vi "FPGA_main_v2.vi"() -> ()   [LabVIEW 2018]
doc: "FPGA main VI for AI input and output.\n\nSamples at 100 kHz and downsamples to 1 kHz."
uses:
  <vilib>/rvi/Emulation/niFpgaGetClockAttributes.vi
  <vilib>/rvi/Emulation/niFpgaSctlEmulationGetInTimedLoop.vi
  <vilib>/rvi/Emulation/niFpgaEmulationReportErrorSimple.vi
  <vilib>/rvi/eio/common/nirviEmuTemplateMethod_errors.vi
  <vilib>/rvi/Emulation/niFpgaEmulationIsFPGAContextNoSignature.vi
  <vilib>/rvi/errors/niFpgaSetErrorForExecOnDevCompSimple.vi
  <vilib>/rvi/eio/common/nirviEmuReportErrorAndStop.vi
  <vilib>/rvi/DataTransferAndStorage/Container/Common/niFpgaContainerGetUniqueNameForEmu.vi
  <vilib>/rvi/FIFO/Fifo_Resource/nirvififoEmulationSetSize.vi
  <vilib>/rvi/FIFO/Fifo_Resource/nirviFifoEmulationQueueMgr.vi
  <instcachedir>/0/nirviFifoEmulationQueueMgr_E5CAEC123FF24DC58D834DCA3CDAA9B5.lvgen/nirviFifoEmulationQueueMgr_E5CAEC123FF24DC58D834DCA3CDAA9B5_003.vi
  <vilib>/rvi/FIFO/Fifo_Resource/nirvififoEmulationDetermineInputValidOut.vi
  <vilib>/rvi/FIFO/Fifo_Resource/nirvififoEmulationCreateLock.vi
  <vilib>/rvi/Emulation/niFpgaProcessEmulError.vi
  <vilib>/rvi/FIFO/Fifo_Resource/nirvififoEmulationObtainLock.vi
  <vilib>/rvi/FIFO/Fifo_Resource/nirvififoEmulationReleaseLock.vi
  <vilib>/rvi/occurrence/nirviWaitOnOccurrenceBase.vi
  <vilib>/rvi/errors/nirviReportUnexpectedCaseInternalError.vi
  <vilib>/rvi/errors/nirviReportUnexpectedCaseInternalError (U32).vi
  <vilib>/rvi/Emulation/niFpgaCriticalErrorInLSC.vi
  <vilib>/Utility/error.llb/Clear Errors.vi
  <vilib>/eio/EIONode/EIONode.xnode
  <vilib>/rvi/DataTransferAndStorage/Container/XNode/niFpgaContainer.xnode
  <vilib>/rvi/FIFO/Fifo_Resource/nirvififoEmulationWrite.vi
  <vilib>/rvi/Analysis/measure/butterworth/XNode/niFpgaButterworthFilter.xnode
  <vilib>/rvi/FIFO/Fifo_Resource/nirvififoEmulationRead.vi
  Components/FPGA functions/FPGA functions.lvlib
panel:
  in  "Count(uSec)":u8=8 caption="I/O sample time (us)"
  out "LPF loop rate (us)":u8
  out "ConnectorC/AI0":fxp<+/-,16,1>
  out "Signal I/O loop rate (us)":u8
  in  "ConnectorC/AO0":i16
  # "Inputs"
  # "Sampling time"
  # "Filtered AI"
  # "For each additional bit of resolution, the signal must be oversampled by a factor of four:\nf_os = 4^w f_s \nwhere w is the number of additional bits of resolution desired, f_s is the original sampling frequency requirement, and f_os is the oversampling frequency\n\nhttp://www.cypress.com/file/236481/download"
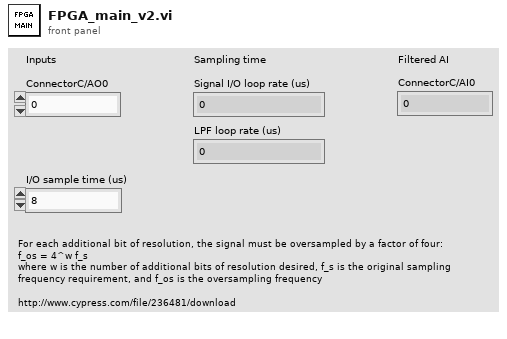
[diagram p1: front panel]
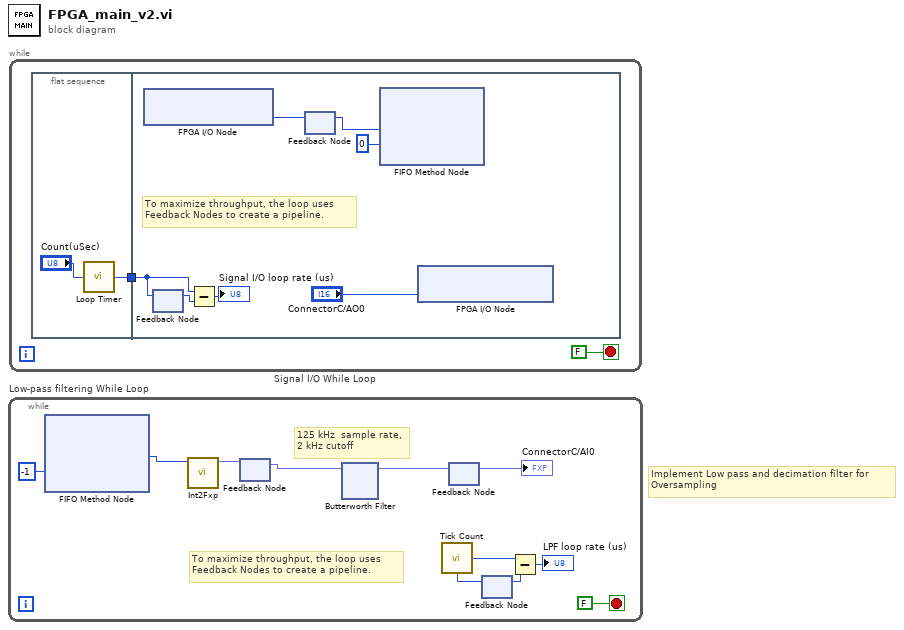
[diagram p0: block diagram]
diagram:
  # "Implement Low pass and decimation filter for \nOversampling"
  n1 = while "Low-pass filtering While Loop" {
    stop <- FALSE stop-if-true
    # "125 kHz  sample rate,\n2 kHz cutoff"
    # "To maximize throughput, the loop uses \nFeedback Nodes to create a pipeline."
    n2 = xnode ("FIFO Method Node")("Timeout"=-1) -> ("Element"=w3:i16)  [unwired: 1 in, 2 out]
    n3 = call "Int2Fxp.vi"("Analog Volt In [Int.]"=w3) -> ("Analog Volt Out [FXP.]"=w2:fxp<+/-,16,1>)  [unwired: 10 in]
    n4 = feedback #1() -> (w1:fxp<+/-,16,1>)  [unwired: 1 in]
    n5 = feedback-in #1(w2) -> ()
    n6 = xnode "Butterworth Filter"("input data"=w1) -> ("output data"=w5:fxp<+/-,16,1>)  [unwired: 2 in]
    n7 = call "Tick Count"() -> ("Tick Count(uSec)"=w8:u8)
    n8 = feedback #2() -> (→"ConnectorC/AI0":fxp<+/-,16,1>)  [unwired: 1 in]
    n9 = feedback-in #2(w5) -> ()
    n10 = feedback-in #3(w8) -> ()
    n11 = feedback #3() -> (w7:u8)  [unwired: 1 in]
    n12 = Subtract(x=w8, y=w7) -> (x-y=→"LPF loop rate (us)":u8)
  }
  n13 = while "Signal I/O While Loop" {
    stop <- FALSE stop-if-true
    n14 = flat-sequence {
      tunnel: [w22] -> w19
      tunnel: w19 -> [w28]
      frame #0 {
        n15 = call "Loop Timer"("Count(uSec)"="Count(uSec)") -> ("Tick Count(uSec)"=w22:u8)
      }
      frame #1 {
        # "To maximize throughput, the loop uses \nFeedback Nodes to create a pipeline."
        n16 = xnode "FPGA I/O Node"() -> ("ConnectorC/AI0"=w26:i16)  [unwired: 1 in, 1 out]
        n17 = feedback #4() -> (w29:u8)  [unwired: 1 in]
        n18 = feedback-in #4(w28) -> ()
        n19 = Subtract(x=w28, y=w29) -> (x-y=→"Signal I/O loop rate (us)":u8)
        n20 = feedback-in #5(w26) -> ()
        n21 = feedback #5() -> (w24:i16)  [unwired: 1 in]
        n22 = xnode ("FIFO Method Node")("Element"=w24, "Timeout"=0) -> ()  [unwired: 1 in, 2 out]
        n23 = xnode "FPGA I/O Node"("ConnectorC/AO0"="ConnectorC/AO0") -> ()  [unwired: 1 in, 1 out]
      }
    }
  }
